vi "AttachThreadInput.vi"(8 "error in (no error)":errorcluster, 9 "Fattach":bool, 10 "threadID attach":u32, 11 "threadID Attachto":u32) -> (0 "error out":errorcluster, 2 "Status":i8)   [LabVIEW 2011]
doc: "SetFocus\nThe SetFocus function sets the keyboard focus to the specified window. The window must be associated with the calling thread's message queue. \n\nHWND SetFocus(\n HWND hWnd // handle to window to receive focus\n);\n \nParameters\nhWnd \nHandle to the window that will receive the keyboard input. If this parameter is NULL, keystrokes are ignored. \nReturn Values\nIf the function succeeds, the return value is the handle to the window that previously had the keyboard focus. If the hWnd parameter is invalid or the window is not associated with the calling thread's message queue, the return value is NULL. To get extended error information, callGetLastError.\n\nRemarks\nThe SetFocus function sends a WM_KILLFOCUS message to the window that loses the keyboard focus and a WM_SETFOCUS message to the window that receives the keyboard focus. It also activates either the window that receives the focus or the parent of the window that receives the focus. \n\nIf a window is active but does not have the focus, any key pressed will produce the WM_SYSCHAR, WM_SYSKEYDOWN, or WM_SYSKEYUP message. If the VK_MENU key is also pressed, the lParam parameter of the message will have bit 30 set. Otherwise, the messages produced do not have this bit set. \n\nBy using the AttachThreadInput function, a thread can attach its input processing to another thread. This allows a thread to call SetFocus to set the keyboard focus to a window associated with another thread's message queue. \n\nWindows CE: Do not use the SetFocus function to set the keyboard focus to a window associated with another thread's message queue. There is one exception. If a window on one thread is the child of the window on the other thread, or if the windows are siblings of the same parent, the thread associated with one window can set the focus to the other window even though it belongs to a different thread. In this case, there is no need to call AttachThreadInput first."
uses:
  user32.dll
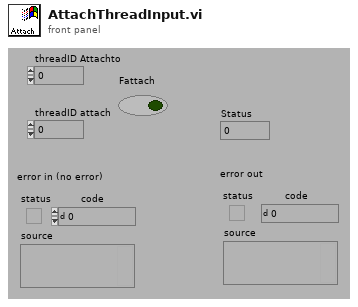
[diagram p1: front panel]
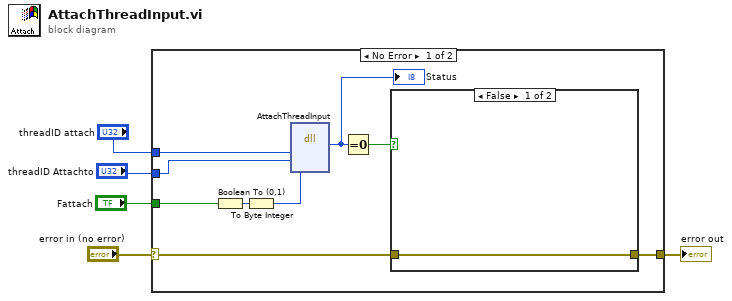
[diagram p0: block diagram]
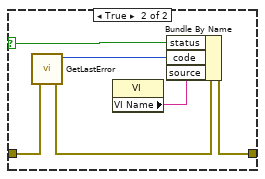
[diagram p2: hidden frame]
diagram:
  n1 = case shown="No Error" "error in (no error)" {
    selector: "error in (no error)" -> [w12 w22]
    tunnel: [w13 w22] -> w5
    tunnel: "threadID attach" -> [w10 _]
    tunnel: "threadID Attachto" -> [w9 _]
    tunnel: "Fattach" -> [w8 _]
    frame No Error {
      n2 = Boolean To (0,1)(Boolean=w8) -> (0, 1=w7:i16)
      n3 = To Byte Integer(number=w7) -> (8bit integer=w6:i8)
      n4 = dll-call lib="user32.dll" fn="AttachThreadInput"("idattach"=w10, "idattachto"=w9, "fattach"=w6) -> ("threadID"=w14:i8)  [unwired: 6 in, 2 out]
      "Status" <- w14
      n5 = Equal To 0?(x=w14) -> (x = 0?=w11:bool)
      n6 = case shown="False" w11 {
        selector: w11 -> [_ w16]
        tunnel: w12 -> [w15 w20]
        tunnel: [w15 w21] -> w13
        frame False {
        }
        frame True {
          n7 = call "GetLastError.vi"("error in (no error)"=w20) -> ("error out"=w19:errorcluster, "CODE"=w18:i32)  [unwired: 5 out]
          n8 = property class="VI"() -> ("VI Name"=w17:string)  [unwired: 2 in, 2 out]
          n9 = Bundle By Name(cluster=w19, "status"=w16, "code"=w18, "source"=w17) -> (w21:errorcluster)
        }
      }
    }
    frame Error {
    }
  }
  "error out" <- w5
